vi "CreateSubVI Parse Plugin Variant.vi"(0 "Create SubVI Variant in":variant) -> (4 "VI has both error in and error out?":bool, 6 "VI Caller Refnum":refnum<vi>)   [LabVIEW 2020]
uses:
  <vilib>/Utility/CreateSubVISupport/CreateSubVI Plugin Data ver1.ctl
  <vilib>/Utility/CreateSubVISupport/CreateSubVI Plugin Data ver2.ctl
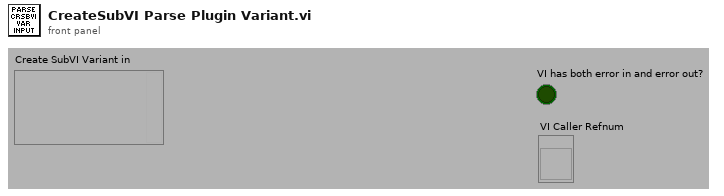
[diagram p1: front panel]
types:
  T1 = typedef "CreateSubVI Plugin Data ver1.ctl" = cluster{"VI has both error in and error out?":bool}
  T2 = typedef "CreateSubVI Plugin Data ver2.ctl" = cluster{"VI has both error in and error out?":bool, "VI Caller Refnum":refnum<vi>}
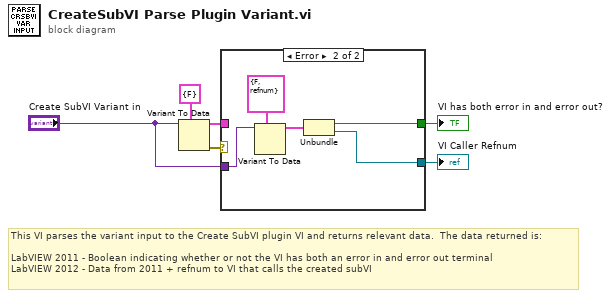
[diagram p0: block diagram]
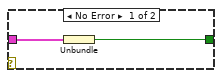
[diagram p2: hidden frame]
diagram:
  # "This VI parses the variant input to the Create SubVI plugin VI and returns relevant data.  The data returned is:\n\nLabVIEW 2011 - Boolean indicating whether or not the VI has both an error in and error out terminal\nLabVIEW 2012 - Data from 2011 + refnum to VI that calls the created subVI"
  n1 = Variant To Data(type=T1 {"VI has both error in and error out?"=FALSE} ("Quick Drop Plugin Data"), Variant="Create SubVI Variant in") -> (data=w6:T1, error out=w3:errorcluster)  [unwired: 1 in]
  n2 = case shown="Error" w3 {
    tunnel: w6 -> [w8 _]
    tunnel: [w7 w10] -> w5
    tunnel: "Create SubVI Variant in" -> [_ w13]
    tunnel: [_ w9] -> w1
    frame No Error {
      n3 = Unbundle(w8) -> ("VI has both error in and error out?"=w7:bool)
    }
    frame Error {
      n4 = Variant To Data(type=T2 {"VI has both error in and error out?"=FALSE, "VI Caller Refnum"=refnum} ("Create SubVI Plugin Data"), Variant=w13) -> (data=w11:T2)  [unwired: 1 in, 1 out]
      n5 = Unbundle(w11) -> ("VI has both error in and error out?"=w10:bool, "VI Caller Refnum"=w9:refnum<vi>)
    }
  }
  "VI has both error in and error out?" <- w5
  "VI Caller Refnum" <- w1
